vi "CoboltLaser_SetpointGet.vi"(0 "ComPort":refnum<visa-resource-name>, 5 "CheckResponse":bool=TRUE, 7 "CurrentModLow":bool, 9 "Mode":T1 caption="Laser Mode", 11 "ErrorIn":errorcluster) -> (4 "ComPortOut":refnum<visa-resource-name>, 6 "Setpoint_Un":dbl format="%.3g", 8 "Setpoint_Pc":dbl, 10 "Response":string, 12 "Units(mW:F)":bool, 13 "MaxSetpoint":dbl, 14 "ResponseOK":bool, 15 "ErrorOut":errorcluster)   [LabVIEW 2019]
doc: "Use this template to build a VI to use as a subVI."
uses:
  Programmes Labview/LabScanV1A/DevicesClass/InstrumentsClass/CoboltMLD/CoboltModes.ctl
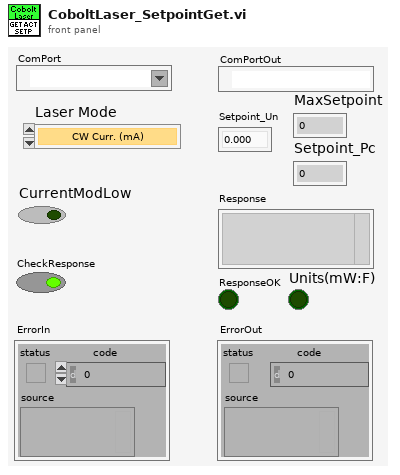
[diagram p1: front panel]
types:
  T1 = typedef "CoboltModes.ctl" = enum16{"CW Curr. (mA)", "CW Pow. (mW)", "Curr. Mod. (mA)", "Pow. Mod. (mW)"}
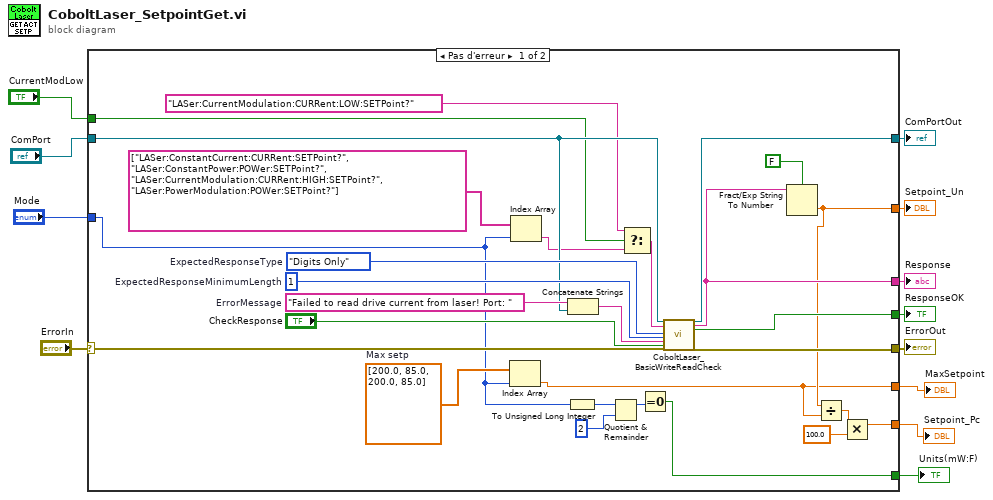
[diagram p0: block diagram]
diagram:
  n1 = case shown="Pas d'erreur" "ErrorIn" {
    selector: "ErrorIn" -> [w40 w42]
    tunnel: [w39 w42] -> w11
    tunnel: "ComPort" -> [w33 w41]
    tunnel: [w32 w41] -> w9
    tunnel: [w22 _] -> w8
    tunnel: [w30 _] -> w7
    tunnel: [w29 _] -> w6
    tunnel: "Mode" -> [w14 _]
    tunnel: "CurrentModLow" -> [w24 _]
    tunnel: [w21 _] -> w3
    tunnel: [w19 _] -> w2
    tunnel: [w13 _] -> w1
    frame No Error {
      w23 = dbl[] [200.0, 85.0, 200.0, 85.0]  # Max setp
      w37 = 1  # ExpectedResponseMinimumLength
      w38 = enum16{"Any", "Digits Only", "Non-Digits Only"}."Digits Only"  # ExpectedResponseType
      w35 = "Failed to read drive current from laser! Port: "  # ErrorMessage
      n2 = Index Array(array=w23, index=w14) -> (element=w21:dbl)
      n3 = Index Array(array=string[] ["LASer:ConstantCurrent:CURRent:SETPoint?", "LASer:ConstantPower:POWer:SETPoint?", "LASer:CurrentModulation:CURRent:HIGH:SETPoint?", "LASer:PowerModulation:POWer:SETPoint?"] ("tableau ajouté"), index=w14) -> (element=w26:string)
      n4 = To Unsigned Long Integer(number=w14) -> (unsigned 32bit integer=w17:u32)
      n5 = Concatenate Strings(w35, w33) -> (w34:string)
      n6 = Quotient & Remainder(x=w17, y=u32 2) -> (x-y*floor(x/y)=w15:u32)  [unwired: 1 out]
      n7 = Select(t="LASer:CurrentModulation:CURRent:LOW:SETPoint?" ("Command"), s=w24, f=w26) -> (s? t:f=w27:string)
      n8 = Equal To 0?(x=w15) -> (x = 0?=w13:bool)
      n9 = call <userlib>:"CoboltLaser_BasicWriteReadCheck.vi"("ComPort"=w33, "Command"=w27, "ExpectedResponseType"=w38, "ExpectedResponseMinimumLength"=w37, "ErrorMessage"=w34, "GenerateError"="CheckResponse", "error in (no error)"=w40) -> ("ComPortOut"=w32:refnum<visa-resource-name>, "Response"=w30:string, "ResponseOK"=w29:bool, "error out"=w39:errorcluster)  [unwired: 17 in]
      n10 = Fract/Exp String To Number(use system decimal point (T)=FALSE, string=w30) -> (number=w22:dbl)  [unwired: 2 in, 1 out]
      n11 = Divide(x=w22, y=w21) -> (x/y=w20:dbl)
      n12 = Multiply(x=w20, y=100.0) -> (x*y=w19:dbl)
    }
    frame Error {
    }
  }
  "ErrorOut" <- w11
  "ComPortOut" <- w9
  "Response" <- w7
  "ResponseOK" <- w6
  "Setpoint_Un" <- w8
  "MaxSetpoint" <- w3
  "Setpoint_Pc" <- w2
  "Units(mW:F)" <- w1
